vi "write_attributes.vi"(8 "error in (no error)":errorcluster, 10 "attributes":T1, 11 "PCA in":refnum<class "PCA.lvclass">) -> (0 "error out":errorcluster, 3 "PCA out":refnum<class "PCA.lvclass">)   [LabVIEW 2020, in "PCA.lvclass"]
uses:
  PCA.lvclass
  Controls/pca_attributes.ctl
  PCA.lvclass/PCA.ctl
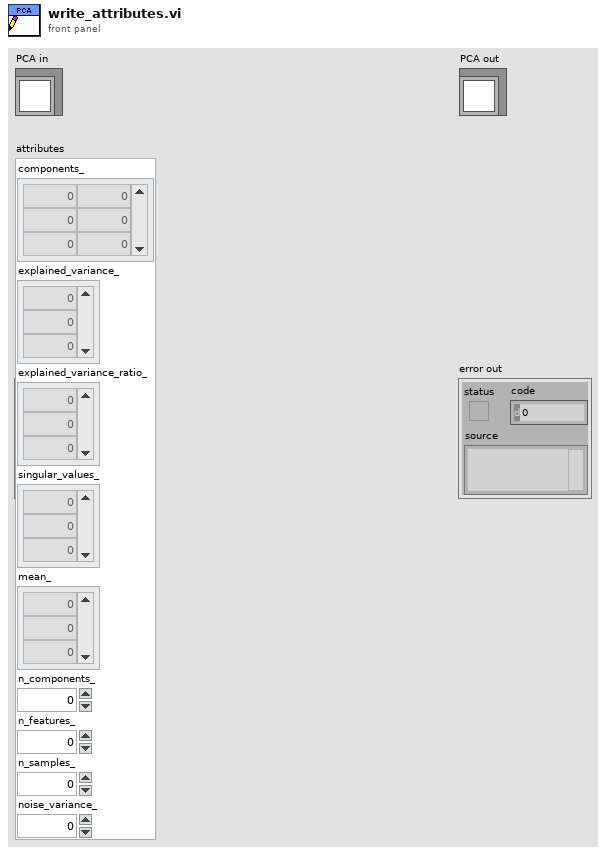
[diagram p1: front panel]
types:
  T1 = typedef "pca_attributes.ctl" = cluster{"components_":dbl[][], "explained_variance_":dbl[], "explained_variance_ratio_":dbl[], "singular_values_":dbl[], "mean_":dbl[], "n_components_":dbl, "n_features_":dbl, "n_samples_":dbl, "noise_variance_":dbl}
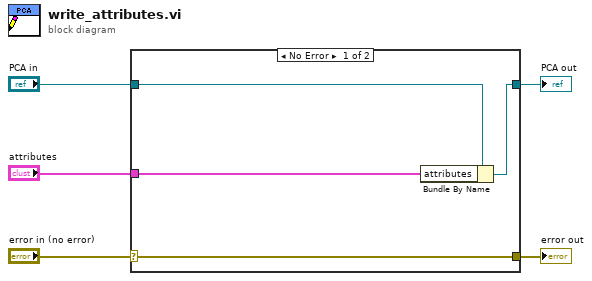
[diagram p0: block diagram]
diagram:
  n1 = case shown="No Error" "error in (no error)" {
    selector: "error in (no error)" -> [w9 w10]
    tunnel: [w9 w10] -> w4
    tunnel: [w7 w11] -> w2
    tunnel: "PCA in" -> [w8 w11]
    tunnel: "attributes" -> [w6 _]
    frame No Error {
      n2 = Bundle By Name(cluster=w8, "attributes"=w6) -> (w7:refnum<class "PCA.lvclass">)
    }
    frame Error {
    }
  }
  "error out" <- w4
  "PCA out" <- w2
